vi "Interest Race_v1.vi"() -> ()   [LabVIEW 2020]
panel:
  in  "milliseconds to wait":u32=15
  out "Interest Accumulated ($)":dbl(graph)=5613.5
  out "Balance ($)":dbl(graph)=561350.0
  out "Interest Accumulated ($)":dbl=5450.0
  in  "Balance ($)":dbl=550450.0
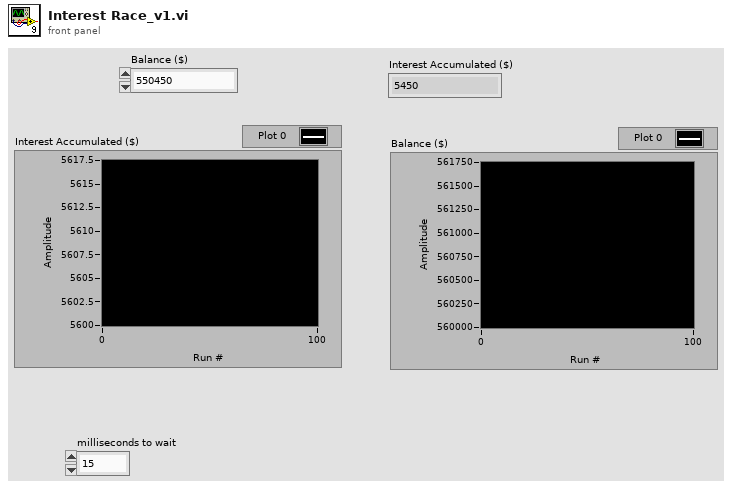
[diagram p1: front panel]
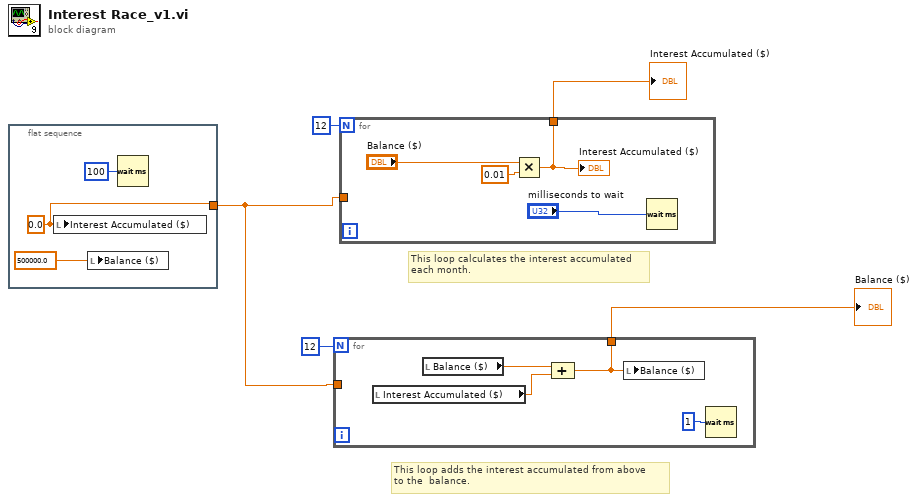
[diagram p0: block diagram]
diagram:
  # "This loop adds the interest accumulated from above\nto the  balance."
  # "This loop calculates the interest accumulated\neach month."
  n1 = flat-sequence {
    tunnel: [w7] -> w3
    frame #0 {
      w7 = 0.0 ("Interest Accumulated ($)")
      n2 = local write "Interest Accumulated ($)"(w7) -> ()
      n3 = local write "Balance ($)"(500000.0 ("Starting Balance ($)")) -> ()
      n4 = Wait (ms)(milliseconds to wait=u32 100) -> ()  [unwired: 1 out]
    }
  }
  n5 = for {
    N: 12 -> [_]
    tunnel: w3 -> [_]
    tunnel: [w9] -> w2
    n6 = local read "Interest Accumulated ($)"() -> (w11:dbl)
    n7 = local read "Balance ($)"() -> (w12:dbl)
    n8 = Compound Arithmetic op=ADD(w12, w11) -> (w9:dbl)
    n9 = local write "Balance ($)"(w9) -> ()
    n10 = Wait (ms)(milliseconds to wait=u32 1) -> ()  [unwired: 1 out]
  }
  "Balance ($)" <- w2
  n11 = for {
    N: 12 -> [_]
    tunnel: w3 -> [_]
    tunnel: [w14] -> w1
    n12 = Multiply(x="Balance ($)", y=0.01) -> (x*y=w14:dbl)
    "Interest Accumulated ($)" <- w14
    n13 = Wait (ms)(milliseconds to wait="milliseconds to wait") -> ()  [unwired: 1 out]
  }
  "Interest Accumulated ($)" <- w1
